vi "General PID Simulator.vi"() -> ()   [LabVIEW 2022 SP3]
doc: "本范例演示如何仿真通用PID控制器。"
uses:
  <vilib>/addons/control/pid/pid.llb/PID (DBL).vi
  <vilib>/addons/control/pid/NI_PID_pid.lvlib
panel:
  in  "PID控制参数":cluster{"P":dbl, "I":dbl, "D":dbl}
  in  "设定值":dbl
  out "波形图表":cluster{"设备输出":dbl, "设定值":dbl}(graph)
  in  "停止":bool
  # "比例"
  # "积分"
  # "微分"
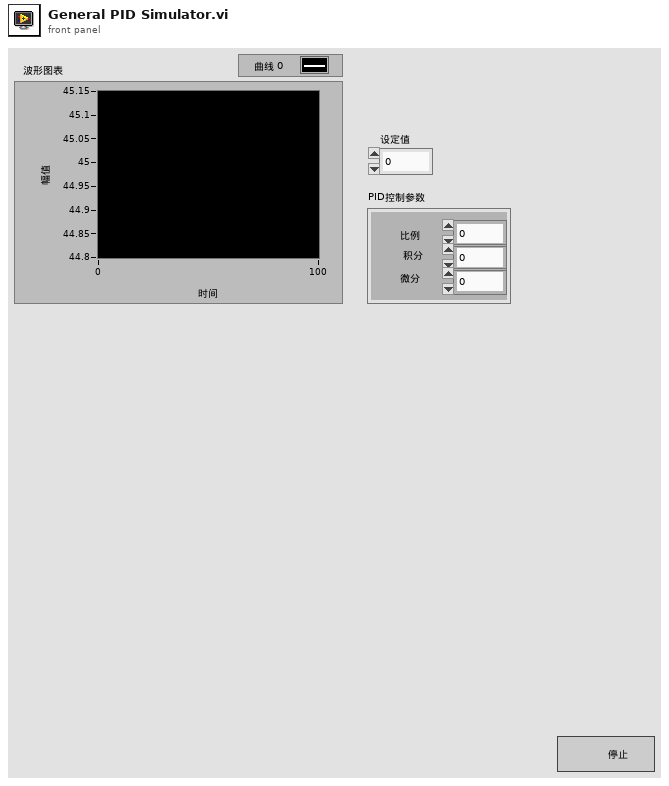
[diagram p1: front panel]
types:
  T1 = cluster{"static gain":dbl, "lag (min)":dbl, "dead cycles":dbl, "load %":dbl, "deadband":dbl, "noise level %":dbl, "initial PV":dbl, "initial PV 2":dbl}
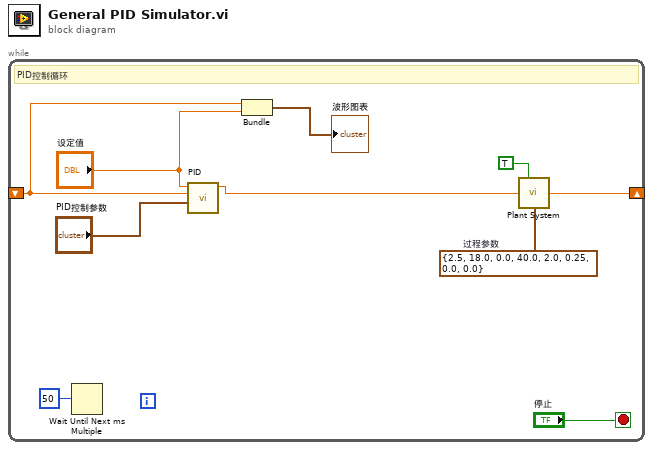
[diagram p0: block diagram]
diagram:
  n1 = while {
    shift-left: _ -> [w9]
    shift-right: [w10] -> _
    stop <- "停止" stop-if-true
    w6 = T1 {"static gain"=2.5, "lag (min)"=18.0, "dead cycles"=0.0, "load %"=40.0, "deadband"=2.0, "noise level %"=0.25, "initial PV"=0.0, "initial PV 2"=0.0}  # 过程参数
    # "PID控制循环"
    n2 = Wait Until Next ms Multiple(millisecond multiple=u32 50 ("unsigned 32bit integer")) -> ()  [unwired: 1 out]
    n3 = call-poly <vilib>:"PID.vi"("PID gains"="PID控制参数", "process variable"=w9, "setpoint"="设定值") -> ("output"=w3:dbl)  [unwired: 7 in, 1 out]
    n4 = Bundle("设备输出"=w9, "设定值"="设定值") -> (→"波形图表":cluster{"设备输出":dbl, "设定值":dbl})  [unwired: 1 in]
    n5 = call "Plant System.vi"("积分器？"=TRUE ("Integrator ?"), "设备输入"=w3, "过程参数"=w6) -> ("设备输出"=w10:dbl)  [unwired: 12 in]
  }
